vi "Image Processing with Vision Assistant (FPGA) -TEST.vi"() -> ()   [LabVIEW 2016]
uses:
  <vilib>/visionFPGA/Controls/IMAQ FPGA Image Size.ctl
  <vilib>/rvi/Emulation/niFpgaSctlEmulationGetInTimedLoop.vi
  <vilib>/rvi/Emulation/niFpgaProcessEmulError.vi
  <vilib>/rvi/Emulation/niFpgaGetClockAttributes.vi
  <vilib>/rvi/Emulation/niFpgaEmulationReportErrorSimple.vi
  <vilib>/visionFPGA/Basics/FIFO to Pixel Bus/IMAQ FPGA FIFO to Pixel Bus RGB32x1.vi
  <vilib>/rvi/eio/common/nirviEmuTemplateMethod_errors.vi
  <vilib>/rvi/DataTransferAndStorage/Container/Common/niFpgaContainerGetUniqueNameForEmu.vi
  <vilib>/rvi/DataTransferAndStorage/Container/Common/niFpgaContainerSetEmuInfo.vi
  <vilib>/rvi/eio/common/nirviEmuReportErrorAndStop.vi
  <vilib>/rvi/interface/RandomDataEmulation/niFpgaRandomDataHandleErrors.vi
  <vilib>/rvi/Emulation/niFpgaCriticalErrorInLSC.vi
  <vilib>/eio/EIONode/EIONode.xnode
  <vilib>/rvi/LocalResourceManager/LocalResourceManager.xnode
  <vilib>/rvi/DataTransferAndStorage/Container/XNode/niFpgaContainer.xnode
  <vilib>/rvi/interface/RandomDataEmulation/nirviRandomDataFpgaReadWriteTemplate.vi
  <vilib>/visionFPGA/NI_VDM_FPGA_Basics.lvlib
panel:
  out "Out Row":u16
  out "Out Col":u16
  out "DV Row":u16
  out "DV Col":u16
  out "Col":u16
  out "Row":u16
  out "Gaussian Out1":u32
  out "In":u32
  out "Comm LED Status":bool=TRUE
  out "Radio LED Status":bool=TRUE
  out "outputExtreme2":bool=TRUE
  out "outputExtreme1":bool=TRUE
  out "outputDOG2":bool=TRUE
  out "outputDOG1":bool=TRUE
  out "outputGaussian2":bool=TRUE
  out "outputGaussian1":bool=TRUE
  out "Output Valid":bool
  out "Ready For Output":bool=TRUE
  out "StartOfImage":bool=TRUE
  in  "Image Size":T1={"Width"=640, "Height"=480}
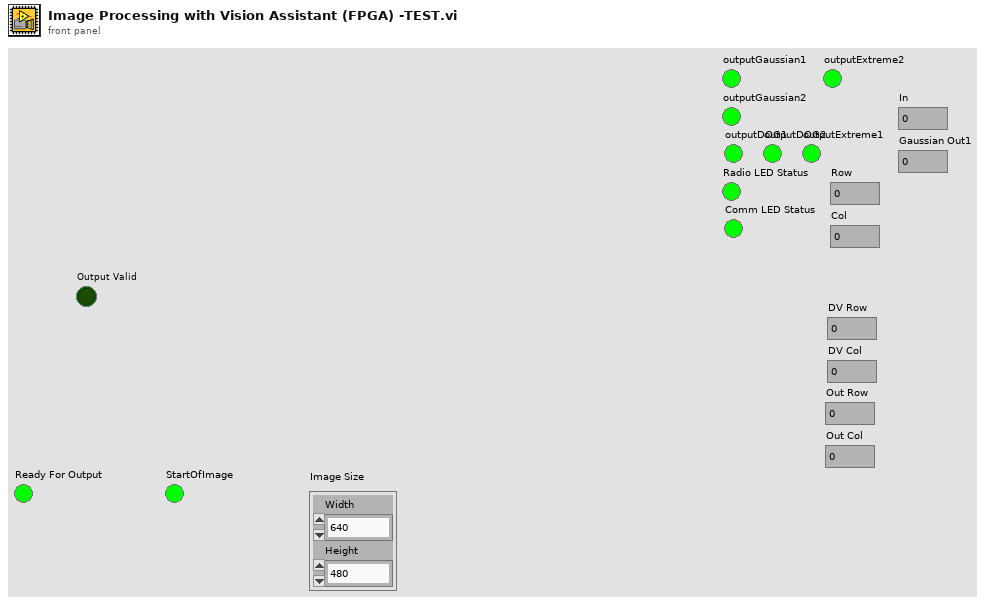
[diagram p1: front panel]
types:
  T1 = typedef "IMAQ FPGA Image Size.ctl" = cluster{"Width":u32, "Height":u32}
  T2 = typedef "IMAQ FPGA Pixel Bus RGB32x1.ctl" = cluster{"Pixel Data":cluster{"A":u8, "R/H":u8, "G/S":u8, "B/L":u8}, "DV":bool, "EOL":bool, "EOI":bool, "Data Type":enum16{"RGB32 x 1"}}
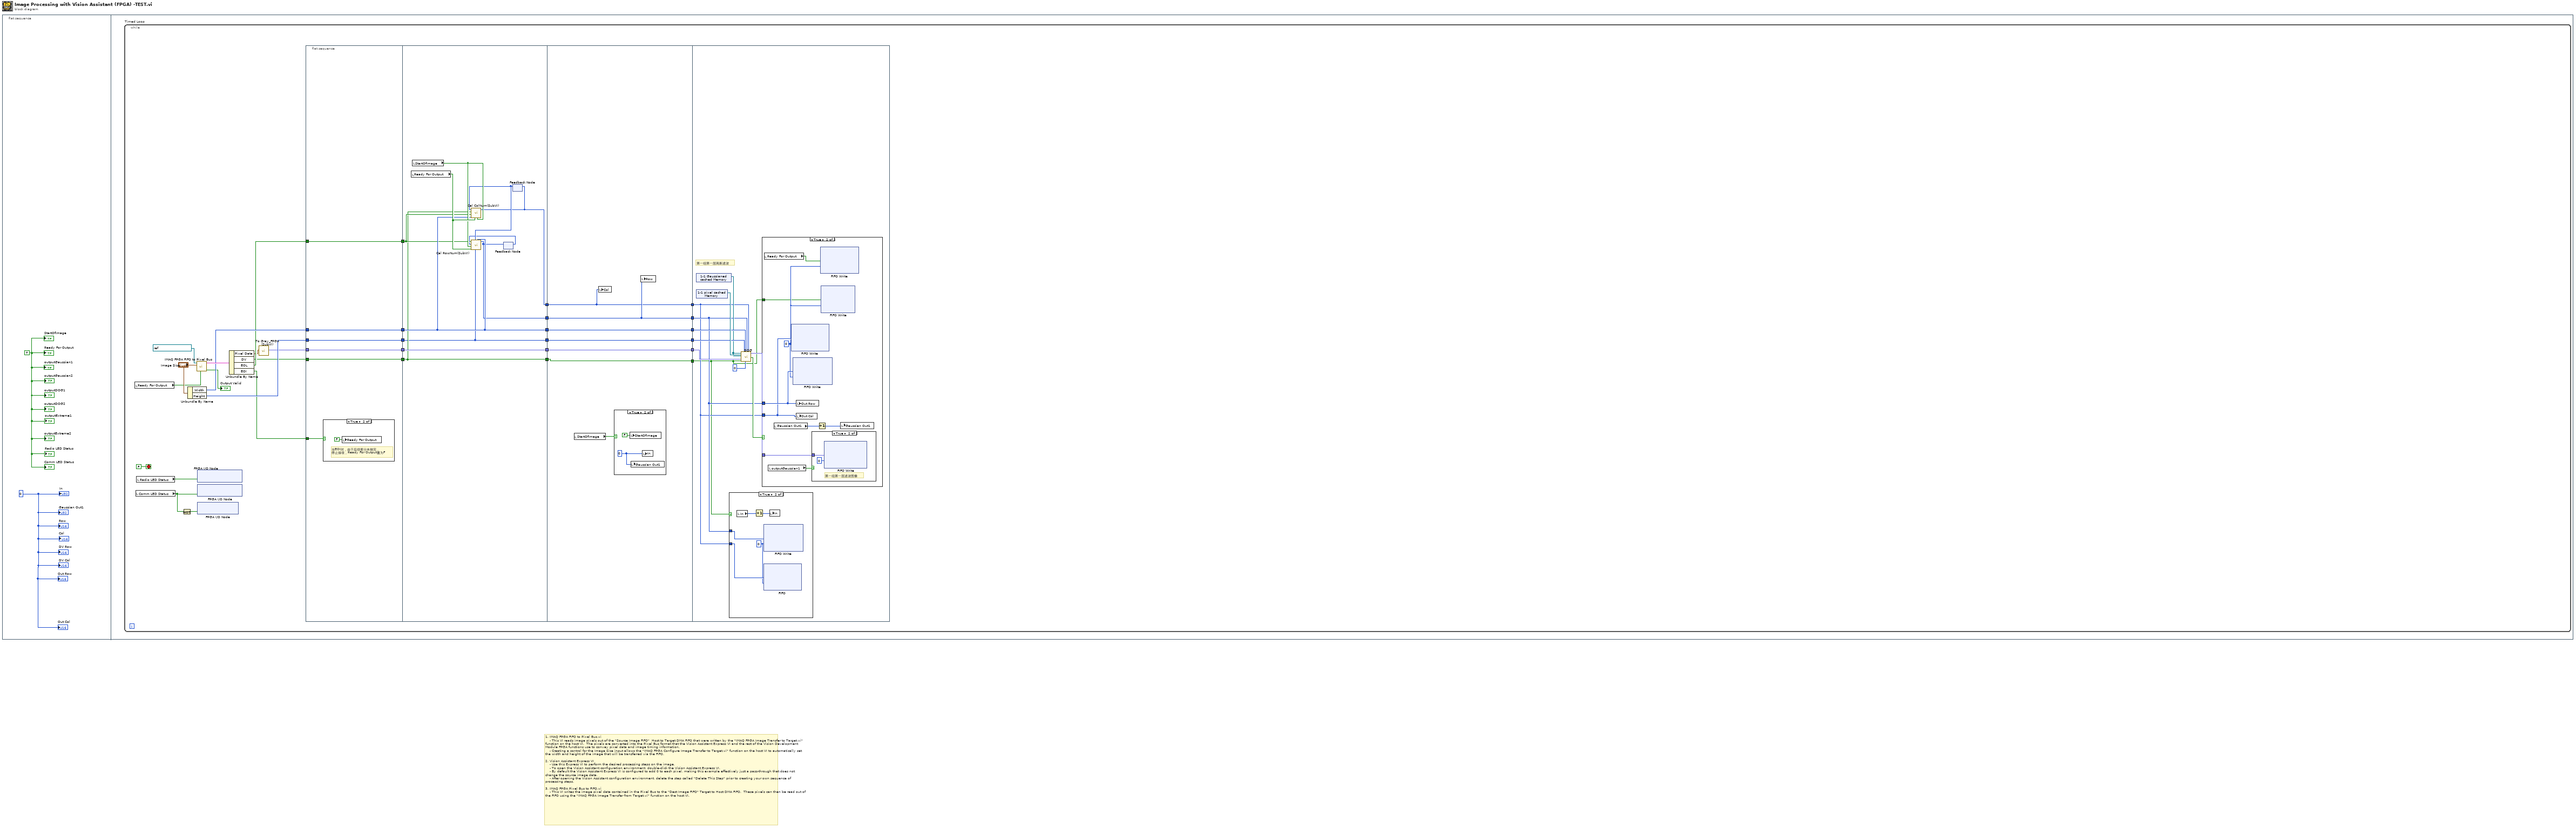
[diagram p0: block diagram]
diagram:
  # "1. IMAQ FPGA FIFO to Pixel Bus.vi\n    - This VI reads image pixels out of the \"Source Image FIFO\"  Host to Target DMA FIFO that were written by the \"IMAQ FPGA Image Transfer to Target.vi\" function on the host VI.  The pixels are converted into the Pixel Bus format that the Vision Assistant Express VI and the rest of the Vision Development Module FPGA functions use to convey pixel data and image timing information.\n    - Creating a control for the Image Size input allows the \"IMAQ FPGA Configure Image Transfer to Target.vi\" function on the host VI to automatically set the width and height of the image that will be transferred via the FIFO.\n\n2. Vision Assistant Express VI\n    - Use this Express VI to perform the desired processing steps on the image.\n    - To open the Vision Assistant configuration environment, double-click the Vision Assistant Express VI.\n    - By default the Vision Assistant Express VI is configured to add 0 to each pixel, making this example effectively just a pass-through that does not change the source image data.\n    - After opening the Vision Assistant configuration environment, delete the step called \"Delete This Step\" prior to creating your own sequence of processing steps.\n\n3. IMAQ FPGA Pixel Bus to FIFO.vi\n    - This VI writes the image pixel data contained in the Pixel Bus to the \"Dest Image FIFO\" Target to Host DMA FIFO.  These pixels can then be read out of the FIFO using the \"IMAQ FPGA Image Transfer from Target.vi\" function on the host VI."
  n1 = flat-sequence {
    frame #0 {
      w1 = i16 0
      w2 = TRUE ("Ready For Output")
      "StartOfImage" <- w2
      "Ready For Output" <- w2
      "outputGaussian1" <- w2
      "outputGaussian2" <- w2
      "outputDOG1" <- w2
      "outputDOG2" <- w2
      "outputExtreme1" <- w2
      "outputExtreme2" <- w2
      "Radio LED Status" <- w2
      "Comm LED Status" <- w2
      "In" <- w1
      "Gaussian Out1" <- w1
      "Row" <- w1
      "Col" <- w1
      "DV Row" <- w1
      "DV Col" <- w1
      "Out Row" <- w1
      "Out Col" <- w1
    }
    frame #1 {
      n2 = while "Timed Loop" {
        stop <- FALSE stop-if-true
        n3 = local read "Ready For Output"() -> (w16:bool)
        n4 = local read "Comm LED Status"() -> (w3:bool)
        n5 = local read "Radio LED Status"() -> (w5:bool)
        n6 = Not(x=w3) -> (.not. x?=w4:bool)
        n7 = Unbundle By Name("Image Size") -> ("Width"=w24:u32, "Height"=w32:u32)
        n8 = call-poly <vilib>:"IMAQ FPGA FIFO to Pixel Bus.vi"("Ready For Output"=w16, "Image Size"="Image Size", "Source Image FIFO"=refnum<k21> "32it Source FIFO") -> ("Output Valid"=→"Output Valid":bool, "Pixel Bus Out"=w34:T2)  [unwired: 6 in, 1 out]
        n9 = xnode "FPGA I/O Node"("Radio LED Green"=w5) -> ()  [unwired: 1 in, 1 out]
        n10 = xnode "FPGA I/O Node"("Mode LED Green"=w3) -> ()  [unwired: 1 in, 1 out]
        n11 = xnode "FPGA I/O Node"("Mode LED Red"=w4) -> ()  [unwired: 1 in, 1 out]
        n12 = Unbundle By Name(w34) -> ("Pixel Data"=w7:cluster{"A":u8, "R/H":u8, "G/S":u8, "B/L":u8}, "DV"=w6:bool, "EOL"=w17:bool, "EOI"=w31:bool)
        n13 = call "To Gray_FPGA (SubVI).vi"("Pixel Data"=w7) -> ("Data Out"=w8:fxp<+,8,8>)  [unwired: 10 in]
        n14 = flat-sequence {
          tunnel: w17 -> [w37]
          tunnel: w31 -> [w36]
          tunnel: w6 -> [w38]
          tunnel: w32 -> [w39]
          tunnel: w24 -> [w40]
          tunnel: w8 -> [w41]
          tunnel: [w41] -> w15
          tunnel: [w40] -> w14
          tunnel: [w39] -> w13
          tunnel: [w38] -> w12
          tunnel: [w37] -> w11
          tunnel: [w45] -> w23
          tunnel: [w43] -> w22
          tunnel: [w53] -> w21
          tunnel: [w50] -> w20
          tunnel: [w47] -> w19
          tunnel: [w48] -> w18
          tunnel: w15 -> [w53]
          tunnel: w14 -> [w50]
          tunnel: w13 -> [w47]
          tunnel: w12 -> [w48]
          tunnel: w11 -> [w49]
          tunnel: [w56] -> w30
          tunnel: [w60] -> w29
          tunnel: [w58] -> w28
          tunnel: [w59] -> w27
          tunnel: [w54] -> w26
          tunnel: [w55] -> w25
          tunnel: w23 -> [w55]
          tunnel: w22 -> [w54]
          tunnel: w21 -> [w60]
          tunnel: w20 -> [w59]
          tunnel: w19 -> [w58]
          tunnel: w18 -> [w56]
          tunnel: w30 -> [w63]
          tunnel: w29 -> [w73]
          tunnel: w28 -> [w69]
          tunnel: w27 -> [w70]
          tunnel: w26 -> [w64]
          tunnel: w25 -> [w65]
          frame #0 {
            n15 = case shown="True" w36 {
              frame False {
              }
              frame True {
                # "当EOI时，由于后续差分未做完，\n停止接收，Ready For Output置为F"
                n16 = local write "Ready For Output"(FALSE ("Ready For Output")) -> ()
              }
            }
          }
          frame #1 {
            n17 = local read "Ready For Output"() -> (w52:bool)
            n18 = local read "StartOfImage"() -> (w51:bool)
            n19 = feedback #1() -> (w44:u16)  [unwired: 1 in]
            n20 = feedback #2() -> (w46:u16)  [unwired: 1 in]
            n21 = call "Cal ColNum(SubVI).vi"("StartOfImage"=w51, "Ready For Input"=w52, "Width"=w50, "EOL"=w49, "DV"=w48, "curColNum"=w46) -> ("nextColNum"=w43:u16)  [unwired: 5 in]
            n22 = call "Cal RowNum(SubVI).vi"("Width"=w50, "Height"=w47, "curCol"=w46, "Ready For Input"=w52, "startOfImage"=w51, "curRow"=w44, "EOL"=w49) -> ("nextRow"=w45:u16)  [unwired: 4 in]
            n23 = feedback-in #1(w45) -> ()
            n24 = feedback-in #2(w43) -> ()
          }
          frame #2 {
            n25 = local read "StartOfImage"() -> (w57:bool)
            n26 = local write "Col"(w54) -> ()
            n27 = case shown="True" w57 {
              frame False {
              }
              frame True {
                w61 = u32 0 ("In")
                n28 = local write "StartOfImage"(FALSE ("StartOfImage")) -> ()
                n29 = local write "Gaussian Out1"(w61) -> ()
                n30 = local write "In"(w61) -> ()
              }
            }
            n31 = local write "Row"(w55) -> ()
          }
          frame #3 {
            # "第一组第一层高斯滤波"
            n32 = xnode "1-1 Gaussianed cached Memory"() -> ("Memory Out"=w67:refnum<k21>)
            n33 = xnode "1-1 pixel cached Memory"() -> ("Memory Out"=w71:refnum<k21>)
            n34 = case shown="True" w63 {
              tunnel: w65 -> [_ w76]
              tunnel: w64 -> [_ w75]
              frame False {
              }
              frame True {
                w74 = 0 ("Timeout")
                n35 = local read "In"() -> (w78:u32)
                n36 = Increment(x=w78) -> (x+1=w77:u32)
                n37 = xnode "FIFO Write"("Element"=w76, "Timeout"=w74) -> ()  [unwired: 1 in, 2 out]
                n38 = xnode "FIFO"("Element"=w75, "Timeout"=w74) -> ()  [unwired: 1 in, 2 out]
                n39 = local write "In"(w77) -> ()
              }
            }
            n40 = call "DOG.vi"("Gaussianed cached Memory"=w67, "pixel cached Memory"=w71, "preGaussianed cached Memory"=w67, "Data in"=w73, "DV in"=w63, "Height"=w69, "Width"=w70, "DelayRowCount"=i16 0, "Rows"=w65, "Cols"=w64) -> ("GaussianFilterData out"=w72:fxp<+,12,12>, "DV out"=w66:bool)  [unwired: 6 in, 2 out]
            n41 = case shown="True" w66 {
              tunnel: w72 -> [_ w87]
              tunnel: w65 -> [_ w83]
              tunnel: w64 -> [_ w82]
              tunnel: w63 -> [_ w79]
              frame False {
              }
              frame True {
                w81 = 0 ("Timeout")
                n42 = local read "Ready For Output"() -> (w80:bool)
                n43 = local read "outputGaussian1"() -> (w86:bool)
                n44 = local read "Gaussian Out1"() -> (w84:u32)
                n45 = xnode ("FIFO Write")("Element"=w82, "Timeout"=w81) -> ()  [unwired: 1 in, 2 out]
                n46 = xnode ("FIFO Write")("Element"=w83, "Timeout"=w81) -> ()  [unwired: 1 in, 2 out]
                n47 = local write "Out Row"(w83) -> ()
                n48 = local write "Out Col"(w82) -> ()
                n49 = case shown="True" w86 {
                  tunnel: w87 -> [_ w88]
                  frame False {
                  }
                  frame True {
                    # "第一组第一层滤波图像"
                    n50 = xnode ("FIFO Write")("Element"=w88, "Timeout"=0) -> ()  [unwired: 1 in, 2 out]
                  }
                }
                n51 = Increment(x=w84) -> (x+1=w85:u32)
                n52 = xnode "FIFO Write"("Element"=w80, "Timeout"=w81) -> ()  [unwired: 1 in, 2 out]
                n53 = xnode "FIFO Write"("Element"=w79, "Timeout"=w81) -> ()  [unwired: 1 in, 2 out]
                n54 = local write "Gaussian Out1"(w85) -> ()
              }
            }
          }
        }
      }
    }
  }
